vi "File.Rotate.Delete Older Files and Folders.vi"(8 "error in":errorcluster, 11 "Task":T1) -> (0 "error out":errorcluster, 3 "Task Out":T1)   [LabVIEW 2024, in "EQMF.lvlib" / "File Utils.lvlib" / "File.Rotate.lvclass"]
uses:
  File.Rotate.lvclass
  File.Rotate.Rotation Task Item.ctl
  File Utils.lvlib
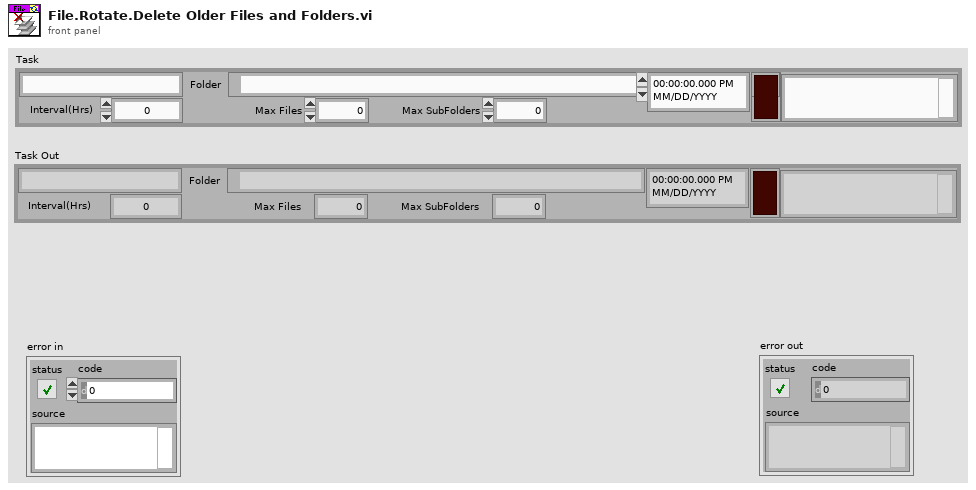
[diagram p1: front panel]
types:
  T1 = typedef "EQMF.lvlib/File Utils.lvlib/File.Rotate.lvclass/File.Rotate.Rotation Task Item.ctl" = cluster{"Name":string, "Interval":dbl, "Folder":path, "Max Files":i32, "Max SubFolders":i32, "LastRotate":timestamp, "Error":bool, "Status":string}
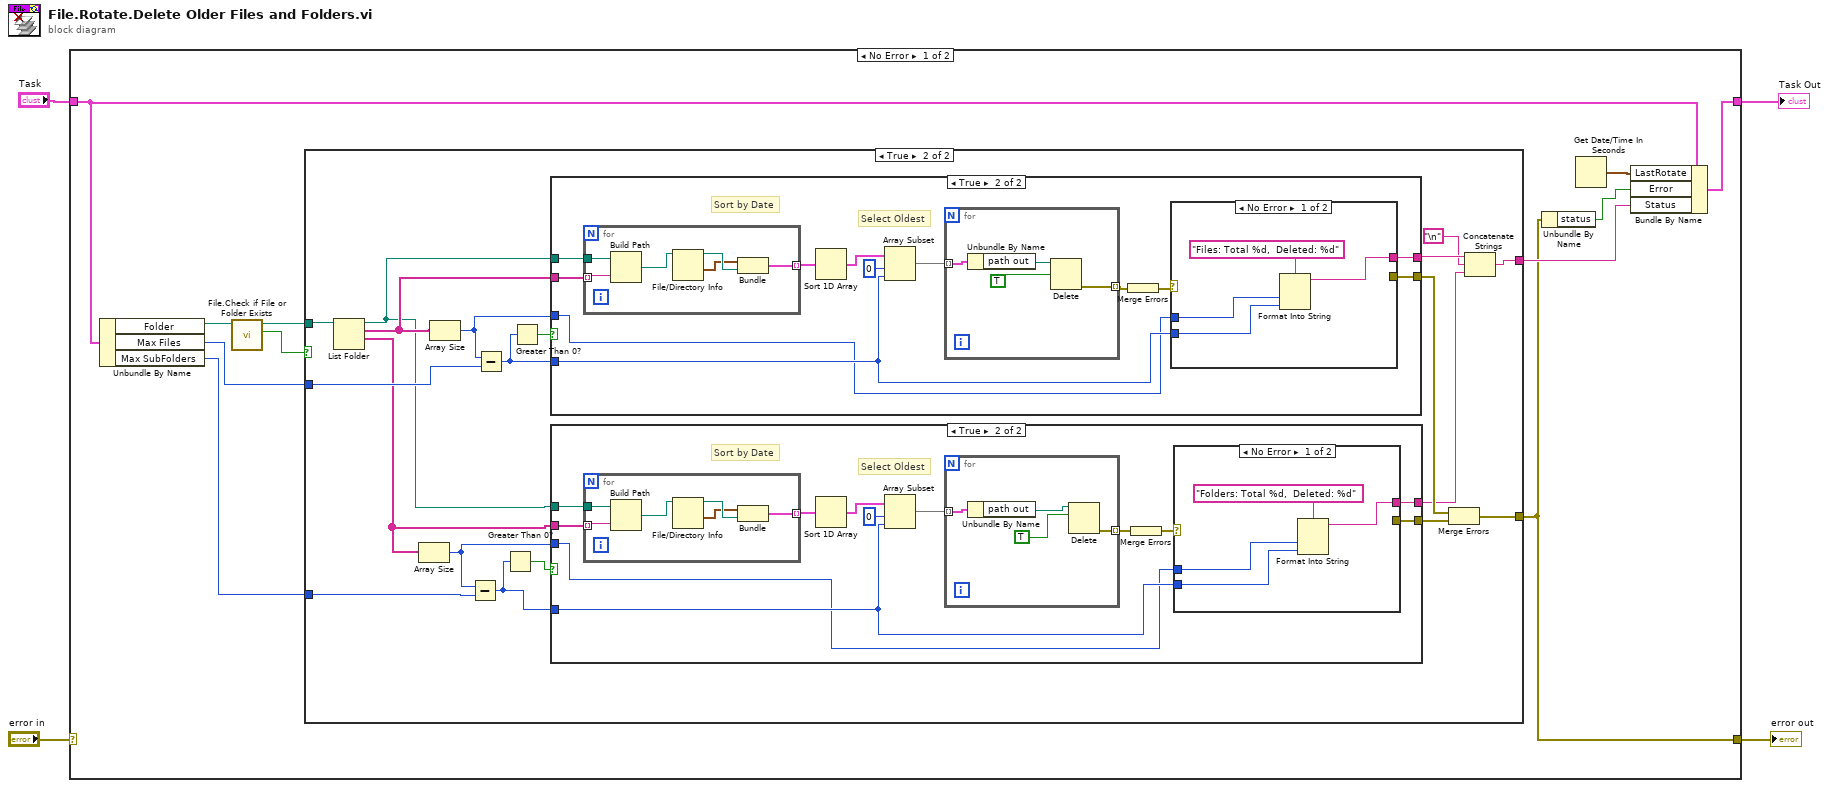
[diagram p0: block diagram]
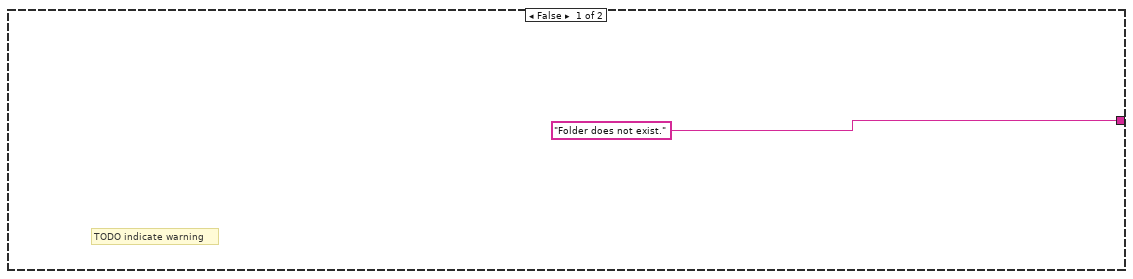
[diagram p2: hidden frame]
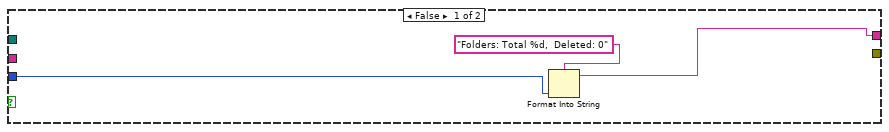
[diagram p3: hidden frame]
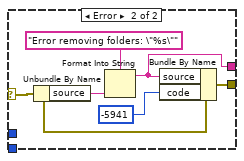
[diagram p4: hidden frame]
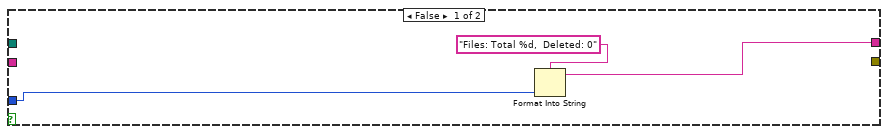
[diagram p5: hidden frame]
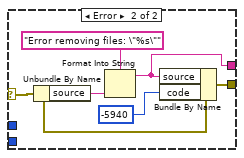
[diagram p6: hidden frame]
diagram:
  n1 = case shown="No Error" "error in" {
    selector: "error in" -> [_ w106]
    tunnel: "Task" -> [w10 w107]
    tunnel: [w9 w107] -> w3
    tunnel: [w5 w106] -> w2
    frame No Error {
      n2 = Unbundle By Name(w10) -> ("Folder"=w15:path, "Max Files"=w12:i32, "Max SubFolders"=w11:i32)
      n3 = call "File.Check if File or Folder Exists.vi"("Path"=w15) -> ("Exists"=w13:bool, "Dup Path"=w14:path)  [unwired: 6 in, 3 out]
      n4 = case shown="True" w13 {
        tunnel: w14 -> [_ w35]
        tunnel: w12 -> [_ w30]
        tunnel: w11 -> [_ w33]
        tunnel: [_ w23] -> w5
        tunnel: ["Folder does not exist." w19] -> w7
        frame False {
          # "TODO indicate warning"
        }
        frame True {
          n5 = List Folder(path=w35) -> (path out=w29:path, filenames=w34:string[], folder names=w28:string[])  [unwired: 3 in, 1 out]
          n6 = Array Size(array=w28) -> (size(s)=w22:i32)
          n7 = Array Size(array=w34) -> (size(s)=w21:i32)
          n8 = Subtract(x=w22, y=w33) -> (x-y=w26:i32)
          n9 = Subtract(x=w21, y=w30) -> (x-y=w31:i32)
          n10 = Greater Than 0?(x=w26) -> (x > 0?=w27:bool)
          n11 = Greater Than 0?(x=w31) -> (x > 0?=w32:bool)
          n12 = case shown="True" w32 {
            tunnel: w29 -> [_ w85]
            tunnel: w34 -> [_ w84]
            tunnel: w31 -> [_ w76]
            tunnel: [_ w77] -> w24
            tunnel: w21 -> [w72 w75]
            tunnel: [w71 w74] -> w20
            frame False {
              n13 = Format Into String(format string="Files: Total %d,  Deleted: 0", w72) -> (resulting string=w71:string)  [unwired: 2 in, 1 out]
            }
            frame True {
              # "Select Oldest"
              # "Sort by Date"
              n14 = for {
                tunnel: w85 -> [w105]
                tunnel: w84 -> [w104] mode=indexing
                tunnel: [w100] -> w83 mode=indexing
                n15 = Build Path(base path=w105, name or relative path=w104) -> (appended path=w103:path)
                n16 = File/Directory Info(path=w103) -> (path out=w102:path, last mod=w101:timestamp)  [unwired: 1 in, 5 out]
                n17 = Bundle("last mod"=w101, "path out"=w102) -> (w100:cluster{"last mod":timestamp, "path out":path})  [unwired: 1 in]
              }
              n18 = Sort 1D Array(array=w83) -> (sorted array=w82:cluster{"last mod":timestamp, "path out":path}[])
              n19 = Array Subset(array=w82, index=0, length=w76) -> (w80:cluster{"last mod":timestamp, "path out":path}[])
              n20 = for {
                tunnel: w80 -> [w99] mode=indexing
                tunnel: [w97] -> w79 mode=indexing
                n21 = Unbundle By Name(w99) -> ("path out"=w98:path)
                n22 = Delete(path (use dialog)=w98, entire hierarchy (F)=TRUE) -> (error out=w97:errorcluster)  [unwired: 3 in, 2 out]
              }
              n23 = Merge Errors(w79) -> (w78:errorcluster)
              n24 = case shown="No Error" w78 {
                selector: w78 -> [_ w93]
                tunnel: [_ w91] -> w77
                tunnel: w76 -> [w88 _]
                tunnel: w75 -> [w87 _]
                tunnel: [w86 w90] -> w74
                frame No Error {
                  n25 = Format Into String(format string="Files: Total %d,  Deleted: %d", w87, w88) -> (resulting string=w86:string)  [unwired: 2 in, 1 out]
                }
                frame Error {
                  n26 = Unbundle By Name(w93) -> ("source"=w94:string)
                  n27 = Format Into String(format string="Error removing files: \"%s\"", w94) -> (resulting string=w90:string)  [unwired: 2 in, 1 out]
                  n28 = Bundle By Name(cluster=w93, "source"=w90, "code"=-5940) -> (w91:errorcluster)
                }
              }
            }
          }
          n29 = case shown="True" w27 {
            tunnel: w29 -> [_ w50]
            tunnel: w28 -> [_ w49]
            tunnel: w26 -> [_ w41]
            tunnel: [_ w42] -> w25
            tunnel: w22 -> [w37 w40]
            tunnel: [w36 w39] -> w18
            frame False {
              n30 = Format Into String(format string="Folders: Total %d,  Deleted: 0", w37) -> (resulting string=w36:string)  [unwired: 2 in, 1 out]
            }
            frame True {
              # "Select Oldest"
              # "Sort by Date"
              n31 = for {
                tunnel: w50 -> [w70]
                tunnel: w49 -> [w69] mode=indexing
                tunnel: [w65] -> w48 mode=indexing
                n32 = Build Path(base path=w70, name or relative path=w69) -> (appended path=w68:path)
                n33 = File/Directory Info(path=w68) -> (path out=w67:path, last mod=w66:timestamp)  [unwired: 1 in, 5 out]
                n34 = Bundle("last mod"=w66, "path out"=w67) -> (w65:cluster{"last mod":timestamp, "path out":path})  [unwired: 1 in]
              }
              n35 = Sort 1D Array(array=w48) -> (sorted array=w47:cluster{"last mod":timestamp, "path out":path}[])
              n36 = Array Subset(array=w47, index=0, length=w41) -> (w45:cluster{"last mod":timestamp, "path out":path}[])
              n37 = for {
                tunnel: w45 -> [w64] mode=indexing
                tunnel: [w61] -> w44 mode=indexing
                n38 = Unbundle By Name(w64) -> ("path out"=w63:path)
                n39 = Delete(path (use dialog)=w63, entire hierarchy (F)=TRUE) -> (error out=w61:errorcluster)  [unwired: 3 in, 2 out]
              }
              n40 = Merge Errors(w44) -> (w43:errorcluster)
              n41 = case shown="No Error" w43 {
                selector: w43 -> [_ w58]
                tunnel: [_ w56] -> w42
                tunnel: w41 -> [w53 _]
                tunnel: w40 -> [w52 _]
                tunnel: [w51 w55] -> w39
                frame No Error {
                  n42 = Format Into String(format string="Folders: Total %d,  Deleted: %d", w52, w53) -> (resulting string=w51:string)  [unwired: 2 in, 1 out]
                }
                frame Error {
                  n43 = Unbundle By Name(w58) -> ("source"=w59:string)
                  n44 = Format Into String(format string="Error removing folders: \"%s\"", w59) -> (resulting string=w55:string)  [unwired: 2 in, 1 out]
                  n45 = Bundle By Name(cluster=w58, "source"=w55, "code"=-5941) -> (w56:errorcluster)
                }
              }
            }
          }
          n46 = Merge Errors(w24, w25) -> (w23:errorcluster)
          n47 = Concatenate Strings(w20, "\n", w18) -> (w19:string)
        }
      }
      n48 = Unbundle By Name(w5) -> ("status"=w6:bool)
      n49 = Get Date/Time In Seconds() -> (seconds since 1Jan1904=w8:timestamp)
      n50 = Bundle By Name(cluster=w10, "LastRotate"=w8, "Error"=w6, "Status"=w7) -> (w9:T1)
    }
    frame Error {
    }
  }
  "error out" <- w2
  "Task Out" <- w3
